vi "S2C_FPGA_Target2TargetFIFO.vi"   [LabVIEW 2015]
uses:
  <vilib>/rvi/DataTransferAndStorage/Container/XNode/niFpgaContainer.xnode
  <vilib>/rvi/FIFO/Fifo_Resource/nirvififoEmulationGetNumberOfElementsToRead.vi
  <vilib>/rvi/FIFO/Fifo_Resource/nirvififoEmulationRead.vi
  <vilib>/eio/EIONode/EIONode.xnode
  <vilib>/rvi/eio/common/nirviEmuTemplateMethod_errors.vi
  S2C_FPGA_Global.vi
types:
  T1 = enum8{"Unknown", "Port_0", "Port_1", "Port_2", "Port_3", "Port_4"}
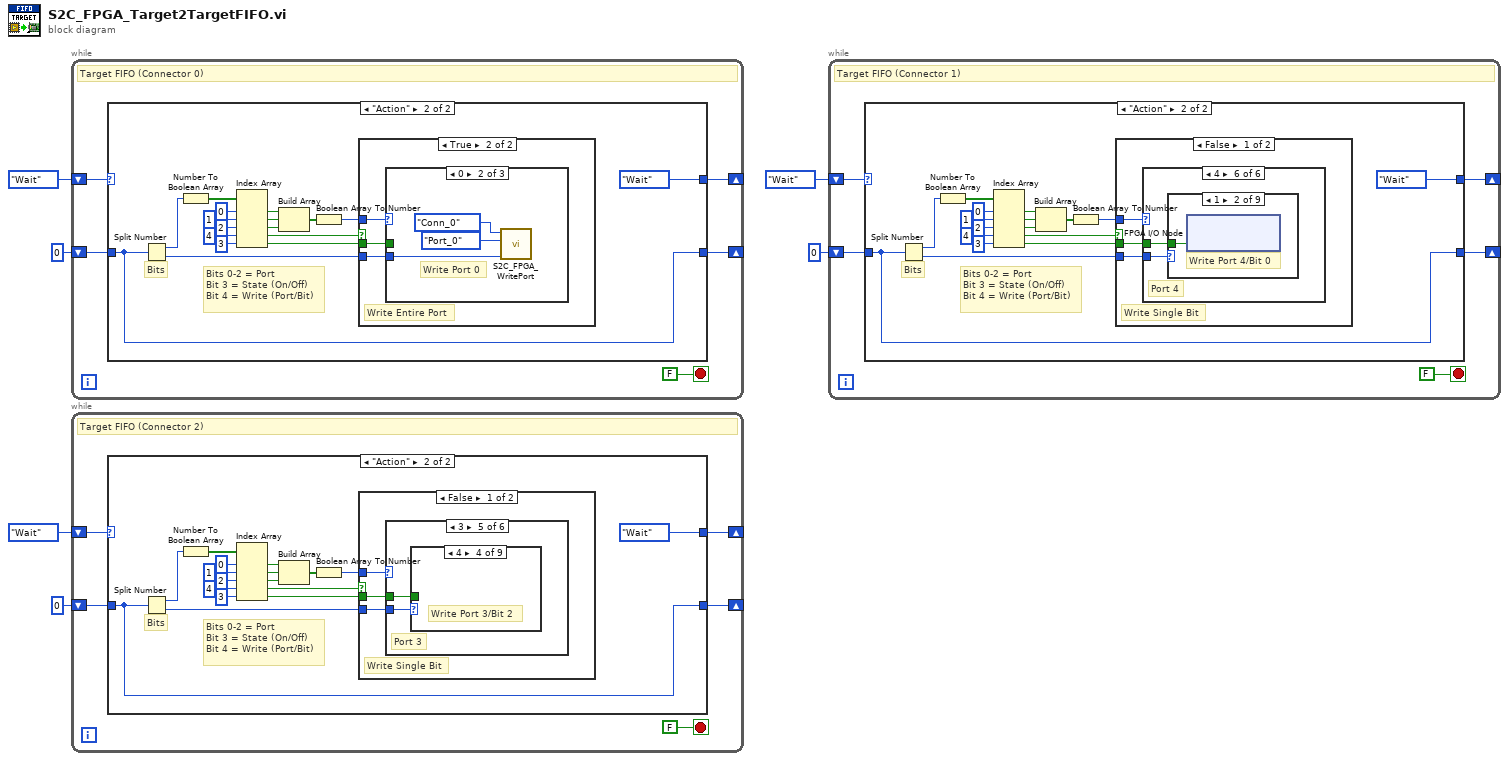
[diagram p0: block diagram]
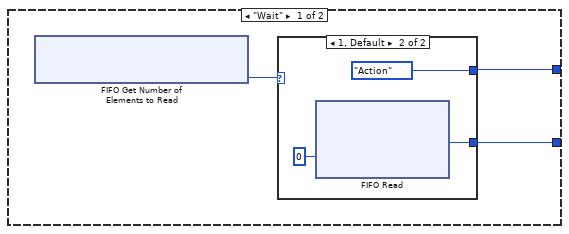
[diagram p2: hidden frame]
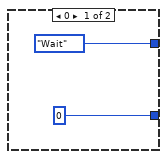
[diagram p3: hidden frame]
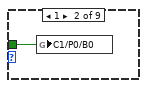
[diagram p6: hidden frame]
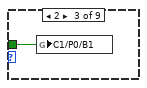
[diagram p7: hidden frame]
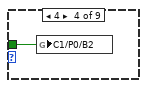
[diagram p8: hidden frame]
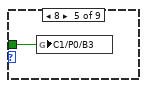
[diagram p9: hidden frame]
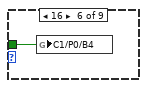
[diagram p10: hidden frame]
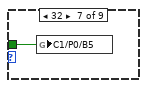
[diagram p11: hidden frame]
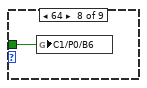
[diagram p12: hidden frame]
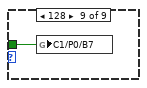
[diagram p13: hidden frame]
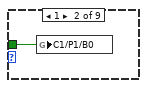
[diagram p15: hidden frame]
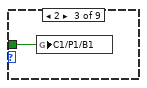
[diagram p16: hidden frame]
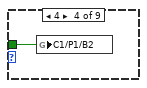
[diagram p17: hidden frame]
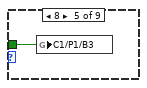
[diagram p18: hidden frame]
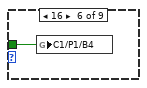
[diagram p19: hidden frame]
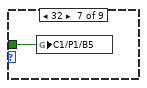
[diagram p20: hidden frame]
diagram:
  n1 = while {
    shift-right: [w10] -> _
    shift-left: enum16{"Wait", "Action"}."Wait" -> [w11]
    shift-right: [w9] -> _
    shift-left: u16 0 ("Element") -> [w8]
    stop <- FALSE stop-if-true
    # "Target FIFO (Connector 0)"
    n2 = case shown="\"Action\"" w11 {
      tunnel: [w13 enum16{"Wait", "Action"}."Wait"] -> w10
      tunnel: [w12 w35] -> w9
      tunnel: w8 -> [_ w35]
      frame "Wait" {
        n3 = xnode ("FIFO Get Number of Elements to Read")() -> ("Number of Elements to Read"=w14:u32)  [unwired: 1 in, 1 out]
        n4 = case shown="1, Default" w14 {
          tunnel: [enum16{"Wait", "Action"}."Wait" enum16{"Wait", "Action"}."Action"] -> w13
          tunnel: [u16 0 ("Element") w18] -> w12
          frame 0 {
          }
          frame 1, Default {
            n5 = xnode ("FIFO Read")("Timeout"=0) -> ("Element"=w18:u16)  [unwired: 1 in, 2 out]
          }
        }
      }
      frame "Action" {
        # "Bits 0-2 = Port\nBit 3 = State (On/Off)\nBit 4 = Write (Port/Bit)"
        # "Bits"
        n6 = Split Number(x=w35) -> (hi(x)=w26:u8, lo(x)=w24:u8)
        n7 = Number To Boolean Array(number=w26) -> (Boolean array=w34:bool[])
        n8 = Index Array(array=w34, index #1=0 ("index"), index #2=1 ("index"), index #3=2 ("index"), index #4=4 ("index"), index #5=3 ("index")) -> (element #1=w31:bool, element #2=w30:bool, element #3=w20:bool, element #4=w21:bool, element #5=w22:bool)
        n9 = Build Array(w31, w30, w20) -> (w29:bool[])
        n10 = Boolean Array To Number(Boolean array=w29) -> (number=w25:u8)
        n11 = case shown="True" w21 {
          tunnel: w25 -> [w39 w52]
          tunnel: w24 -> [w38 w51]
          tunnel: w22 -> [w37 w50]
          frame False {
            # "Write Single Bit"
            n12 = case shown="1" w39 {
              tunnel: w38 -> [_ w41 w48]
              tunnel: w37 -> [_ w40 w47]
              frame 5, Default {
              }
              frame 0 {
                # "Port 0"
                n13 = case shown="128" w41 {
                  tunnel: w40 -> [_ w42 w43 w44 _ _ _ w45 w46]
                  frame 0, Default {
                  }
                  frame 1 {
                    # "Write Port 0/Bit 0"
                    n14 = xnode "FPGA I/O Node"("C0/P0/B0"=w42) -> ()  [unwired: 1 in, 1 out]
                  }
                  frame 2 {
                    # "Write Port 0/Bit 1"
                    n15 = xnode "FPGA I/O Node"("C0/P0/B1"=w43) -> ()  [unwired: 1 in, 1 out]
                  }
                  frame 4 {
                    # "Write Port 0/Bit 2"
                    n16 = xnode "FPGA I/O Node"("C0/P0/B2"=w44) -> ()  [unwired: 1 in, 1 out]
                  }
                  frame 8 {
                    # "Write Port 0/Bit 3"
                  }
                  frame 16 {
                    # "Write Port 0/Bit 4"
                  }
                  frame 32 {
                    # "Write Port 0/Bit 5"
                  }
                  frame 64 {
                    # "Write Port 0/Bit 6"
                    n17 = xnode "FPGA I/O Node"("C0/P0/B6"=w45) -> ()  [unwired: 1 in, 1 out]
                  }
                  frame 128 {
                    # "Write Port 0/Bit 7"
                    n18 = xnode "FPGA I/O Node"("C0/P0/B7"=w46) -> ()  [unwired: 1 in, 1 out]
                  }
                }
              }
              frame 1 {
                # "Port 1"
                n19 = case shown="128" w48 {
                  tunnel: w47 -> [_ w49 _ _ _ _ _ _ _]
                  frame 0, Default {
                  }
                  frame 1 {
                    # "Write Port 1/Bit 0"
                    n20 = xnode "FPGA I/O Node"("C0/P1/B0"=w49) -> ()  [unwired: 1 in, 1 out]
                  }
                  frame 2 {
                    # "Write Port 1/Bit 1"
                  }
                  frame 4 {
                    # "Write Port 1/Bit 2"
                  }
                  frame 8 {
                    # "Write Port 1/Bit 3"
                  }
                  frame 16 {
                    # "Write Port 1/Bit 4"
                  }
                  frame 32 {
                    # "Write Port 1/Bit 5"
                  }
                  frame 64 {
                    # "Write Port 1/Bit 6"
                  }
                  frame 128 {
                    # "Write Port 1/Bit 7"
                  }
                }
              }
            }
          }
          frame True {
            # "Write Entire Port"
            n21 = case shown="0" w52 {
              tunnel: w51 -> [_ w53 w56]
              tunnel: w50 -> [_ _ _]
              frame 5, Default {
              }
              frame 0 {
                # "Write Port 0"
                n22 = call "S2C_FPGA_WritePort.vi"("Data"=w53, "Port"=T1."Port_0", "Connector"=enum8{"Conn_0", "Conn_1", "Conn_2"}."Conn_0") -> ()  [unwired: 9 in]
              }
              frame 1 {
                # "Write Port 1"
                n23 = call "S2C_FPGA_WritePort.vi"("Data"=w56, "Port"=T1."Port_1", "Connector"=enum8{"Conn_0", "Conn_1", "Conn_2"}."Conn_0") -> ()  [unwired: 9 in]
              }
            }
          }
        }
      }
    }
  }
  n24 = while {
    shift-right: [w62] -> _
    shift-left: enum16{"Wait", "Action"}."Wait" -> [w63]
    shift-right: [w61] -> _
    shift-left: u16 0 ("Element") -> [w60]
    stop <- FALSE stop-if-true
    # "Target FIFO (Connector 2)"
    n25 = case shown="\"Action\"" w63 {
      tunnel: [w65 enum16{"Wait", "Action"}."Wait"] -> w62
      tunnel: [w64 w87] -> w61
      tunnel: w60 -> [_ w87]
      frame "Wait" {
        n26 = xnode ("FIFO Get Number of Elements to Read")() -> ("Number of Elements to Read"=w66:u32)  [unwired: 1 in, 1 out]
        n27 = case shown="1, Default" w66 {
          tunnel: [enum16{"Wait", "Action"}."Wait" enum16{"Wait", "Action"}."Action"] -> w65
          tunnel: [u16 0 ("Element") w70] -> w64
          frame 0 {
          }
          frame 1, Default {
            n28 = xnode ("FIFO Read")("Timeout"=0) -> ("Element"=w70:u16)  [unwired: 1 in, 2 out]
          }
        }
      }
      frame "Action" {
        # "Bits 0-2 = Port\nBit 3 = State (On/Off)\nBit 4 = Write (Port/Bit)"
        # "Bits"
        n29 = Split Number(x=w87) -> (hi(x)=w78:u8, lo(x)=w76:u8)
        n30 = Number To Boolean Array(number=w78) -> (Boolean array=w86:bool[])
        n31 = Index Array(array=w86, index #1=0 ("index"), index #2=1 ("index"), index #3=2 ("index"), index #4=4 ("index"), index #5=3 ("index")) -> (element #1=w83:bool, element #2=w82:bool, element #3=w72:bool, element #4=w73:bool, element #5=w74:bool)
        n32 = Build Array(w83, w82, w72) -> (w81:bool[])
        n33 = Boolean Array To Number(Boolean array=w81) -> (number=w77:u8)
        n34 = case shown="False" w73 {
          tunnel: w77 -> [w91 w142]
          tunnel: w76 -> [w90 w141]
          tunnel: w74 -> [w89 w140]
          frame False {
            # "Write Single Bit"
            n35 = case shown="3" w91 {
              tunnel: w90 -> [_ w93 w103 w113 w123 w131]
              tunnel: w89 -> [_ w92 w102 w112 w122 w130]
              frame 5, Default {
              }
              frame 0 {
                # "Port 0"
                n36 = case shown="1" w93 {
                  tunnel: w92 -> [_ w94 w95 w96 w97 w98 w99 w100 w101]
                  frame 0, Default {
                  }
                  frame 1 {
                    # "Write Port 0/Bit 0"
                    n37 = xnode "FPGA I/O Node"("C2/P0/B0"=w94) -> ()  [unwired: 1 in, 1 out]
                  }
                  frame 2 {
                    # "Write Port 0/Bit 1"
                    n38 = xnode "FPGA I/O Node"("C2/P0/B1"=w95) -> ()  [unwired: 1 in, 1 out]
                  }
                  frame 4 {
                    # "Write Port 0/Bit 2"
                    n39 = xnode "FPGA I/O Node"("C2/P0/B2"=w96) -> ()  [unwired: 1 in, 1 out]
                  }
                  frame 8 {
                    # "Write Port 0/Bit 3"
                    n40 = xnode "FPGA I/O Node"("C2/P0/B3"=w97) -> ()  [unwired: 1 in, 1 out]
                  }
                  frame 16 {
                    # "Write Port 0/Bit 4"
                    n41 = xnode "FPGA I/O Node"("C2/P0/B4"=w98) -> ()  [unwired: 1 in, 1 out]
                  }
                  frame 32 {
                    # "Write Port 0/Bit 5"
                    n42 = xnode "FPGA I/O Node"("C2/P0/B5"=w99) -> ()  [unwired: 1 in, 1 out]
                  }
                  frame 64 {
                    # "Write Port 0/Bit 6"
                    n43 = xnode "FPGA I/O Node"("C2/P0/B6"=w100) -> ()  [unwired: 1 in, 1 out]
                  }
                  frame 128 {
                    # "Write Port 0/Bit 7"
                    n44 = xnode "FPGA I/O Node"("C2/P0/B7"=w101) -> ()  [unwired: 1 in, 1 out]
                  }
                }
              }
              frame 1 {
                # "Port 1"
                n45 = case shown="1" w103 {
                  tunnel: w102 -> [_ w104 w105 w106 w107 w108 w109 w110 w111]
                  frame 0, Default {
                  }
                  frame 1 {
                    # "Write Port 1/Bit 0"
                    n46 = xnode "FPGA I/O Node"("C2/P1/B0"=w104) -> ()  [unwired: 1 in, 1 out]
                  }
                  frame 2 {
                    # "Write Port 1/Bit 1"
                    n47 = xnode "FPGA I/O Node"("C2/P1/B1"=w105) -> ()  [unwired: 1 in, 1 out]
                  }
                  frame 4 {
                    # "Write Port 1/Bit 2"
                    n48 = xnode "FPGA I/O Node"("C2/P1/B2"=w106) -> ()  [unwired: 1 in, 1 out]
                  }
                  frame 8 {
                    # "Write Port 1/Bit 3"
                    n49 = xnode "FPGA I/O Node"("C2/P1/B3"=w107) -> ()  [unwired: 1 in, 1 out]
                  }
                  frame 16 {
                    # "Write Port 1/Bit 4"
                    n50 = xnode "FPGA I/O Node"("C2/P1/B4"=w108) -> ()  [unwired: 1 in, 1 out]
                  }
                  frame 32 {
                    # "Write Port 1/Bit 5"
                    n51 = xnode "FPGA I/O Node"("C2/P1/B5"=w109) -> ()  [unwired: 1 in, 1 out]
                  }
                  frame 64 {
                    # "Write Port 1/Bit 6"
                    n52 = xnode "FPGA I/O Node"("C2/P1/B6"=w110) -> ()  [unwired: 1 in, 1 out]
                  }
                  frame 128 {
                    # "Write Port 1/Bit 7"
                    n53 = xnode "FPGA I/O Node"("C2/P1/B7"=w111) -> ()  [unwired: 1 in, 1 out]
                  }
                }
              }
              frame 2 {
                # "Port 2"
                n54 = case shown="128" w113 {
                  tunnel: w112 -> [_ w114 w115 w116 w117 w118 w119 w120 w121]
                  frame 0, Default {
                  }
                  frame 1 {
                    # "Write Port 2/Bit 0"
                    n55 = xnode "FPGA I/O Node"("C2/P2/B0"=w114) -> ()  [unwired: 1 in, 1 out]
                  }
                  frame 2 {
                    # "Write Port 2/Bit 1"
                    n56 = xnode "FPGA I/O Node"("C2/P2/B1"=w115) -> ()  [unwired: 1 in, 1 out]
                  }
                  frame 4 {
                    # "Write Port 2/Bit 2"
                    n57 = xnode "FPGA I/O Node"("C2/P2/B2"=w116) -> ()  [unwired: 1 in, 1 out]
                  }
                  frame 8 {
                    # "Write Port 2/Bit 3"
                    n58 = xnode "FPGA I/O Node"("C2/P2/B3"=w117) -> ()  [unwired: 1 in, 1 out]
                  }
                  frame 16 {
                    # "Write Port 2/Bit 4"
                    n59 = xnode "FPGA I/O Node"("C2/P2/B4"=w118) -> ()  [unwired: 1 in, 1 out]
                  }
                  frame 32 {
                    # "Write Port 2/Bit 5"
                    n60 = xnode "FPGA I/O Node"("C2/P2/B5"=w119) -> ()  [unwired: 1 in, 1 out]
                  }
                  frame 64 {
                    # "Write Port 2/Bit 6"
                    n61 = xnode "FPGA I/O Node"("C2/P2/B6"=w120) -> ()  [unwired: 1 in, 1 out]
                  }
                  frame 128 {
                    # "Write Port 2/Bit 7"
                    n62 = xnode "FPGA I/O Node"("C2/P2/B7"=w121) -> ()  [unwired: 1 in, 1 out]
                  }
                }
              }
              frame 3 {
                # "Port 3"
                n63 = case shown="4" w123 {
                  tunnel: w122 -> [_ _ w124 _ w125 w126 w127 w128 w129]
                  frame 0, Default {
                  }
                  frame 1 {
                    # "Write Port 3/Bit 0"
                  }
                  frame 2 {
                    # "Write Port 3/Bit 1"
                    n64 = xnode "FPGA I/O Node"("C2/P3/B1"=w124) -> ()  [unwired: 1 in, 1 out]
                  }
                  frame 4 {
                    # "Write Port 3/Bit 2"
                  }
                  frame 8 {
                    # "Write Port 3/Bit 3"
                    n65 = xnode "FPGA I/O Node"("C2/P3/B3"=w125) -> ()  [unwired: 1 in, 1 out]
                  }
                  frame 16 {
                    # "Write Port 3/Bit 4"
                    n66 = xnode "FPGA I/O Node"("C2/P3/B4"=w126) -> ()  [unwired: 1 in, 1 out]
                  }
                  frame 32 {
                    # "Write Port 3/Bit 5"
                    n67 = xnode "FPGA I/O Node"("C2/P3/B5"=w127) -> ()  [unwired: 1 in, 1 out]
                  }
                  frame 64 {
                    # "Write Port 3/Bit 6"
                    n68 = xnode "FPGA I/O Node"("C2/P3/B6"=w128) -> ()  [unwired: 1 in, 1 out]
                  }
                  frame 128 {
                    # "Write Port 3/Bit 7"
                    n69 = xnode "FPGA I/O Node"("C2/P3/B7"=w129) -> ()  [unwired: 1 in, 1 out]
                  }
                }
              }
              frame 4 {
                # "Port 4"
                n70 = case shown="4" w131 {
                  tunnel: w130 -> [_ w132 w133 w134 w135 w136 w137 w138 w139]
                  frame 0, Default {
                  }
                  frame 1 {
                    # "Write Port 4/Bit 0"
                    n71 = xnode "FPGA I/O Node"("C2/P4/B0"=w132) -> ()  [unwired: 1 in, 1 out]
                  }
                  frame 2 {
                    # "Write Port 4/Bit 1"
                    n72 = xnode "FPGA I/O Node"("C2/P4/B1"=w133) -> ()  [unwired: 1 in, 1 out]
                  }
                  frame 4 {
                    # "Write Port 4/Bit 2"
                    n73 = xnode "FPGA I/O Node"("C2/P4/B2"=w134) -> ()  [unwired: 1 in, 1 out]
                  }
                  frame 8 {
                    # "Write Port 4/Bit 3"
                    n74 = xnode "FPGA I/O Node"("C2/P4/B3"=w135) -> ()  [unwired: 1 in, 1 out]
                  }
                  frame 16 {
                    # "Write Port 4/Bit 4"
                    n75 = xnode "FPGA I/O Node"("C2/P4/B4"=w136) -> ()  [unwired: 1 in, 1 out]
                  }
                  frame 32 {
                    # "Write Port 4/Bit 5"
                    n76 = xnode "FPGA I/O Node"("C2/P4/B5"=w137) -> ()  [unwired: 1 in, 1 out]
                  }
                  frame 64 {
                    # "Write Port 4/Bit 6"
                    n77 = xnode "FPGA I/O Node"("C2/P4/B6"=w138) -> ()  [unwired: 1 in, 1 out]
                  }
                  frame 128 {
                    # "Write Port 4/Bit 7"
                    n78 = xnode "FPGA I/O Node"("C2/P4/B7"=w139) -> ()  [unwired: 1 in, 1 out]
                  }
                }
              }
            }
          }
          frame True {
            # "Write Entire Port"
            n79 = case shown="0" w142 {
              tunnel: w141 -> [_ w143 w146 w149 w152 w155]
              tunnel: w140 -> [_ _ _ _ _ _]
              frame 5, Default {
              }
              frame 0 {
                # "Write Port 0"
                n80 = call "S2C_FPGA_WritePort.vi"("Data"=w143, "Port"=T1."Port_0", "Connector"=enum8{"Conn_0", "Conn_1", "Conn_2"}."Conn_2") -> ()  [unwired: 9 in]
              }
              frame 1 {
                # "Write Port 1"
                n81 = call "S2C_FPGA_WritePort.vi"("Data"=w146, "Port"=T1."Port_1", "Connector"=enum8{"Conn_0", "Conn_1", "Conn_2"}."Conn_2") -> ()  [unwired: 9 in]
              }
              frame 2 {
                # "Write Port 2"
                n82 = call "S2C_FPGA_WritePort.vi"("Data"=w149, "Port"=T1."Port_2", "Connector"=enum8{"Conn_0", "Conn_1", "Conn_2"}."Conn_2") -> ()  [unwired: 9 in]
              }
              frame 3 {
                # "Write Port 3"
                n83 = call "S2C_FPGA_WritePort.vi"("Data"=w152, "Port"=T1."Port_3", "Connector"=enum8{"Conn_0", "Conn_1", "Conn_2"}."Conn_2") -> ()  [unwired: 9 in]
              }
              frame 4 {
                # "Write Port 4"
                n84 = call "S2C_FPGA_WritePort.vi"("Data"=w155, "Port"=T1."Port_4", "Connector"=enum8{"Conn_0", "Conn_1", "Conn_2"}."Conn_2") -> ()  [unwired: 9 in]
              }
            }
          }
        }
      }
    }
  }
  n85 = while {
    shift-right: [w161] -> _
    shift-left: enum16{"Wait", "Action"}."Wait" -> [w162]
    shift-right: [w160] -> _
    shift-left: u16 0 ("Element") -> [w159]
    stop <- FALSE stop-if-true
    # "Target FIFO (Connector 1)"
    n86 = case shown="\"Action\"" w162 {
      tunnel: [w164 enum16{"Wait", "Action"}."Wait"] -> w161
      tunnel: [w163 w186] -> w160
      tunnel: w159 -> [_ w186]
      frame "Wait" {
        n87 = xnode ("FIFO Get Number of Elements to Read")() -> ("Number of Elements to Read"=w165:u32)  [unwired: 1 in, 1 out]
        n88 = case shown="1, Default" w165 {
          tunnel: [enum16{"Wait", "Action"}."Wait" enum16{"Wait", "Action"}."Action"] -> w164
          tunnel: [u16 0 ("Element") w169] -> w163
          frame 0 {
          }
          frame 1, Default {
            n89 = xnode ("FIFO Read")("Timeout"=0) -> ("Element"=w169:u16)  [unwired: 1 in, 2 out]
          }
        }
      }
      frame "Action" {
        # "Bits 0-2 = Port\nBit 3 = State (On/Off)\nBit 4 = Write (Port/Bit)"
        # "Bits"
        n90 = Split Number(x=w186) -> (hi(x)=w177:u8, lo(x)=w175:u8)
        n91 = Number To Boolean Array(number=w177) -> (Boolean array=w185:bool[])
        n92 = Index Array(array=w185, index #1=0 ("index"), index #2=1 ("index"), index #3=2 ("index"), index #4=4 ("index"), index #5=3 ("index")) -> (element #1=w182:bool, element #2=w181:bool, element #3=w171:bool, element #4=w172:bool, element #5=w173:bool)
        n93 = Build Array(w182, w181, w171) -> (w180:bool[])
        n94 = Boolean Array To Number(Boolean array=w180) -> (number=w176:u8)
        n95 = case shown="False" w172 {
          tunnel: w176 -> [w190 w233]
          tunnel: w175 -> [w189 w232]
          tunnel: w173 -> [w188 w231]
          frame False {
            # "Write Single Bit"
            n96 = case shown="4" w190 {
              tunnel: w189 -> [_ w192 w202 w212 w220 w226]
              tunnel: w188 -> [_ w191 w201 w211 w219 w225]
              frame 5, Default {
              }
              frame 0 {
                # "Port 0"
                n97 = case shown="0, Default" w192 {
                  tunnel: w191 -> [_ w193 w194 w195 w196 w197 w198 w199 w200]
                  frame 0, Default {
                  }
                  frame 1 {
                    n98 = global write "S2C_FPGA_Global.vi" "C1/P0/B0"(w193) -> ()
                  }
                  frame 2 {
                    n99 = global write "S2C_FPGA_Global.vi" "C1/P0/B1"(w194) -> ()
                  }
                  frame 4 {
                    n100 = global write "S2C_FPGA_Global.vi" "C1/P0/B2"(w195) -> ()
                  }
                  frame 8 {
                    n101 = global write "S2C_FPGA_Global.vi" "C1/P0/B3"(w196) -> ()
                  }
                  frame 16 {
                    n102 = global write "S2C_FPGA_Global.vi" "C1/P0/B4"(w197) -> ()
                  }
                  frame 32 {
                    n103 = global write "S2C_FPGA_Global.vi" "C1/P0/B5"(w198) -> ()
                  }
                  frame 64 {
                    n104 = global write "S2C_FPGA_Global.vi" "C1/P0/B6"(w199) -> ()
                  }
                  frame 128 {
                    n105 = global write "S2C_FPGA_Global.vi" "C1/P0/B7"(w200) -> ()
                  }
                }
              }
              frame 1 {
                # "Port 1"
                n106 = case shown="0, Default" w202 {
                  tunnel: w201 -> [_ w203 w204 w205 w206 w207 w208 w209 w210]
                  frame 0, Default {
                  }
                  frame 1 {
                    n107 = global write "S2C_FPGA_Global.vi" "C1/P1/B0"(w203) -> ()
                  }
                  frame 2 {
                    n108 = global write "S2C_FPGA_Global.vi" "C1/P1/B1"(w204) -> ()
                  }
                  frame 4 {
                    n109 = global write "S2C_FPGA_Global.vi" "C1/P1/B2"(w205) -> ()
                  }
                  frame 8 {
                    n110 = global write "S2C_FPGA_Global.vi" "C1/P1/B3"(w206) -> ()
                  }
                  frame 16 {
                    n111 = global write "S2C_FPGA_Global.vi" "C1/P1/B4"(w207) -> ()
                  }
                  frame 32 {
                    n112 = global write "S2C_FPGA_Global.vi" "C1/P1/B5"(w208) -> ()
                  }
                  frame 64 {
                    n113 = global write "S2C_FPGA_Global.vi" "C1/P1/B6"(w209) -> ()
                  }
                  frame 128 {
                    n114 = global write "S2C_FPGA_Global.vi" "C1/P1/B7"(w210) -> ()
                  }
                }
              }
              frame 2 {
                # "Port 2"
                n115 = case shown="128" w212 {
                  tunnel: w211 -> [_ w213 w214 w215 _ w216 w217 w218 _]
                  frame 0, Default {
                  }
                  frame 1 {
                    n116 = global write "S2C_FPGA_Global.vi" "C1/P2/B0"(w213) -> ()
                  }
                  frame 2 {
                    n117 = global write "S2C_FPGA_Global.vi" "C1/P2/B1"(w214) -> ()
                  }
                  frame 4 {
                    # "Write Port 2/Bit 2"
                    n118 = xnode "FPGA I/O Node"("C1/P2/B2"=w215) -> ()  [unwired: 1 in, 1 out]
                  }
                  frame 8 {
                    # "Write Port 2/Bit 3"
                  }
                  frame 16 {
                    n119 = global write "S2C_FPGA_Global.vi" "C1/P2/B4"(w216) -> ()
                  }
                  frame 32 {
                    n120 = global write "S2C_FPGA_Global.vi" "C1/P2/B5"(w217) -> ()
                  }
                  frame 64 {
                    # "Write Port 2/Bit 6"
                    n121 = xnode "FPGA I/O Node"("C1/P2/B6"=w218) -> ()  [unwired: 1 in, 1 out]
                  }
                  frame 128 {
                    # "Write Port 2/Bit 7"
                  }
                }
              }
              frame 3 {
                # "Port 3"
                n122 = case shown="128" w220 {
                  tunnel: w219 -> [_ w221 w222 w223 _ w224 _ _ _]
                  frame 0, Default {
                  }
                  frame 1 {
                    n123 = global write "S2C_FPGA_Global.vi" "C1/P3/B0"(w221) -> ()
                  }
                  frame 2 {
                    n124 = global write "S2C_FPGA_Global.vi" "C1/P3/B1"(w222) -> ()
                  }
                  frame 4 {
                    # "Write Port 3/Bit 2"
                    n125 = xnode "FPGA I/O Node"("C1/P3/B2"=w223) -> ()  [unwired: 1 in, 1 out]
                  }
                  frame 8 {
                    # "Write Port 3/Bit 3"
                  }
                  frame 16 {
                    # "Write Port 3/Bit 4"
                    n126 = xnode "FPGA I/O Node"("C1/P3/B4"=w224) -> ()  [unwired: 1 in, 1 out]
                  }
                  frame 32 {
                    # "Write Port 3/Bit 5"
                  }
                  frame 64 {
                    # "Write Port 3/Bit 6"
                  }
                  frame 128 {
                    # "Write Port 3/Bit 7"
                  }
                }
              }
              frame 4 {
                # "Port 4"
                n127 = case shown="1" w226 {
                  tunnel: w225 -> [_ w227 w228 _ _ w229 w230 _ _]
                  frame 0, Default {
                  }
                  frame 1 {
                    # "Write Port 4/Bit 0"
                    n128 = xnode "FPGA I/O Node"("C1/P4/B0"=w227) -> ()  [unwired: 1 in, 1 out]
                  }
                  frame 2 {
                    # "Write Port 4/Bit 1"
                    n129 = xnode "FPGA I/O Node"("C1/P4/B1"=w228) -> ()  [unwired: 1 in, 1 out]
                  }
                  frame 4 {
                    # "Write Port 4/Bit 2"
                  }
                  frame 8 {
                    # "Write Port 4/Bit 3"
                  }
                  frame 16 {
                    # "Write Port 4/Bit 4"
                    n130 = xnode "FPGA I/O Node"("C1/P4/B4"=w229) -> ()  [unwired: 1 in, 1 out]
                  }
                  frame 32 {
                    # "Write Port 4/Bit 5"
                    n131 = xnode "FPGA I/O Node"("C1/P4/B5"=w230) -> ()  [unwired: 1 in, 1 out]
                  }
                  frame 64 {
                    # "Write Port 4/Bit 6"
                  }
                  frame 128 {
                    # "Write Port 4/Bit 7"
                  }
                }
              }
            }
          }
          frame True {
            # "Write Entire Port"
            n132 = case shown="0" w233 {
              tunnel: w232 -> [_ w234 w237 w240 w243 w246]
              tunnel: w231 -> [_ _ _ _ _ _]
              frame 5, Default {
              }
              frame 0 {
                # "Write Port 0"
                n133 = call "S2C_FPGA_WritePort.vi"("Data"=w234, "Port"=T1."Port_0", "Connector"=enum8{"Conn_0", "Conn_1", "Conn_2"}."Conn_1") -> ()  [unwired: 9 in]
              }
              frame 1 {
                # "Write Port 1"
                n134 = call "S2C_FPGA_WritePort.vi"("Data"=w237, "Port"=T1."Port_1", "Connector"=enum8{"Conn_0", "Conn_1", "Conn_2"}."Conn_1") -> ()  [unwired: 9 in]
              }
              frame 2 {
                # "Write Port 2"
                n135 = call "S2C_FPGA_WritePort.vi"("Data"=w240, "Port"=T1."Port_2", "Connector"=enum8{"Conn_0", "Conn_1", "Conn_2"}."Conn_1") -> ()  [unwired: 9 in]
              }
              frame 3 {
                # "Write Port 3"
                n136 = call "S2C_FPGA_WritePort.vi"("Data"=w243, "Port"=T1."Port_3", "Connector"=enum8{"Conn_0", "Conn_1", "Conn_2"}."Conn_1") -> ()  [unwired: 9 in]
              }
              frame 4 {
                # "Write Port 4"
                n137 = call "S2C_FPGA_WritePort.vi"("Data"=w246, "Port"=T1."Port_4", "Connector"=enum8{"Conn_0", "Conn_1", "Conn_2"}."Conn_1") -> ()  [unwired: 9 in]
              }
            }
          }
        }
      }
    }
  }
